vi "Read Digitizer Setting.vi"(8 "error in (no error)":errorcluster, 11 "Digitizer configuration":refnum<class "Digitizer configuration.lvclass">) -> (0 "error out":errorcluster, 2 "Digitizer Setting":T1={"SampleMode"="", "SampleDuration"=0.0, "SampleRate"=100000, "ReferenceClock"="", "SampleClockEdge"="", "TrigType"="", "TrigLevel"=0.0, "TrigSource"="", "Pretrigger"=0.0, "TrigDest"=""} {"TrigLevel" format="%#_f"; "Pretrigger" format="%#_f"; "SampleRate" format="%#_6p"; "SampleDuration" format="%#_6p"}, 3 "Digitizer configuration out":refnum<class "Digitizer configuration.lvclass">)   [LabVIEW 2025, in "Digitizer.lvlib" / "Digitizer configuration.lvclass"]
uses:
  Digitizer configuration.lvclass
  Digitizer Instrument Setting.ctl
  Digitizer configuration.lvclass/Digitizer configuration.ctl
panel:
  # "Sampling"
  # "Trigger"
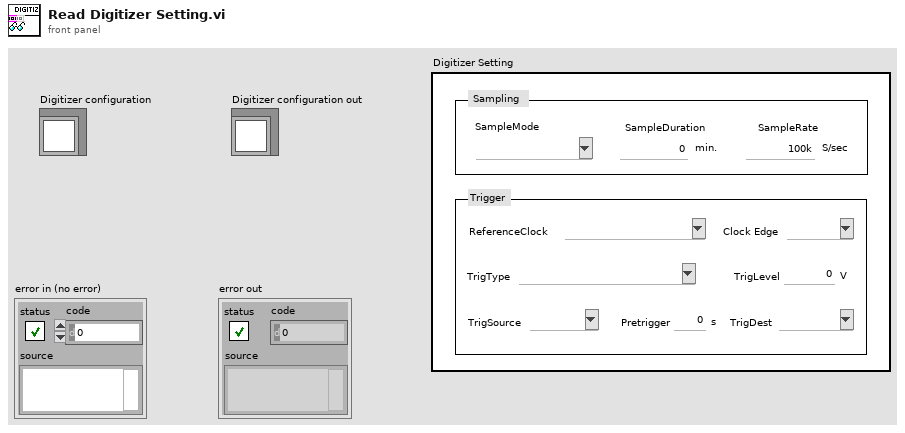
[diagram p1: front panel]
types:
  T1 = typedef "Digitizer.lvlib/Digitizer configuration.lvclass/Digitizer Instrument Setting.ctl" = cluster{"SampleMode":string, "SampleDuration":dbl, "SampleRate":u32, "ReferenceClock":string, "SampleClockEdge":string, "TrigType":string, "TrigLevel":dbl, "TrigSource":string, "Pretrigger":dbl, "TrigDest":string}
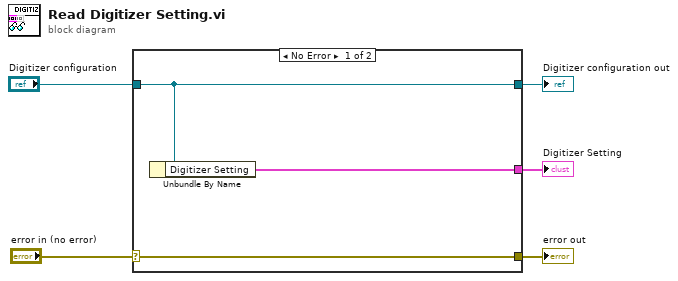
[diagram p0: block diagram]
diagram:
  n1 = case shown="No Error" "error in (no error)" {
    selector: "error in (no error)" -> [w8 w9]
    tunnel: [w8 w9] -> w4
    tunnel: [w7 w10] -> w2
    tunnel: "Digitizer configuration" -> [w7 w10]
    tunnel: [w6 _] -> w1
    frame No Error {
      n2 = Unbundle By Name(w7) -> ("Digitizer Setting"=w6:T1)
    }
    frame Error {
    }
  }
  "error out" <- w4
  "Digitizer configuration out" <- w2
  "Digitizer Setting" <- w1
